vi "HOST.vi"() -> ()   [LabVIEW 2018]
uses:
  <instrlib>/niDMM/nidmm.llb/niDMM Function.ctl
  <instrlib>/niDMM/nidmm.llb/niDMM Resolution in Digits.ctl
  <instrlib>/niDMM/nidmm.llb/niDMM Configure Measurement Digits.vi
panel:
  in  "ЛОГИ":path=path "D:/NI LabVIEW/20.089_(KMKS_2)/LOGS"
  out "T(t)":dbl(graph)=398.0450506439805
  out "3ph P(t)":dbl(graph)
  out "3ph power, V":dbl=2.1649482628491312e-07 format="%#.5f"
  out "Temp, °C":dbl caption="Measurement" format="%.5f"
  out "Amps":dbl caption="Measurement" format="%.5f"
  out "Volts":dbl caption="Measurement" format="%.5f"
  out "Volts (Temp)":dbl caption="Measurement" format="%.5f"
  out "Power, V":dbl=7.216494209497104e-08 format="%#.5f"
  in  "Stop":bool
  in  "Temp Range\n(Volts)":dbl=2.0 format="%.2p"
  out "Out of Range (I)":bool caption="Signal Out of Range"
  in  "I":refnum<k15>="PXI1Slot5"
  in  "Range (Amps)":dbl=1.0 format="%.2p"
  out "Out of Range (V)":bool caption="Signal Out of Range"
  in  "U":refnum<k15>="PXI1Slot4"
  in  "Range (Volts)":dbl=2.0 format="%.2p"
  out "Out of Range (V, Temp)":bool caption="Signal Out of Range"
  in  "Temp":refnum<k15>="PXI1Slot3_4"
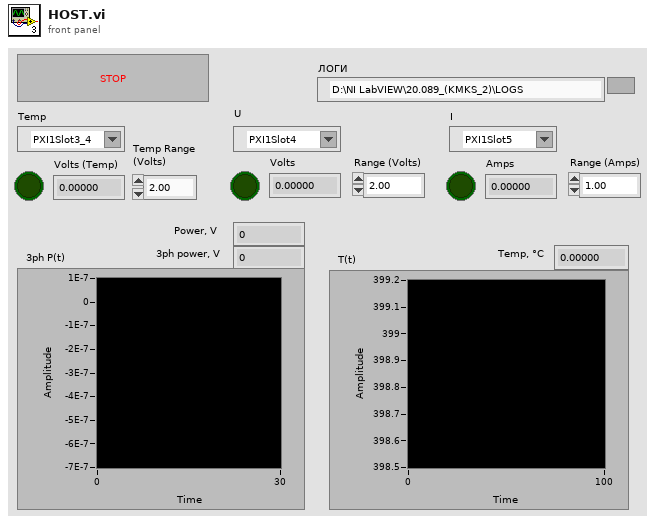
[diagram p1: front panel]
types:
  T1 = enum16{"open", "replace", "create", "open or create", "replace or create", "replace or create with confirmation"}
  T2 = typedef "niDMM Function.ctl" = enum16{"DC Volts", "AC Volts", "DC Current", "AC Current", "2-wire Resistance", "4-wire Resistance", "Diode", "Frequency", "Period", "AC Volts DC Coupled", "Capacitance", "Inductance", "Temperature"}
  T3 = typedef "niDMM Resolution in Digits.ctl" = dbl
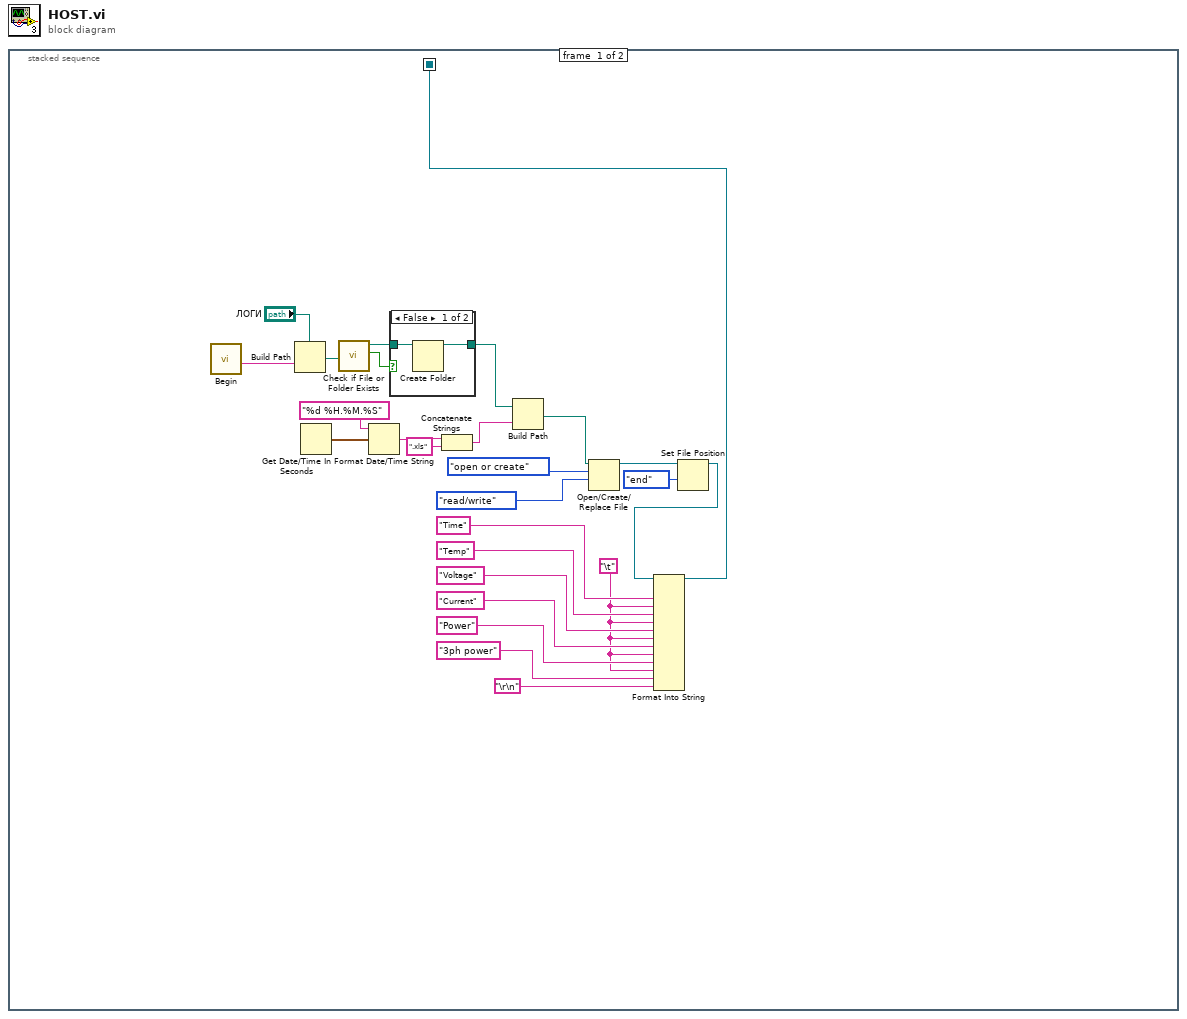
[diagram p0: block diagram]
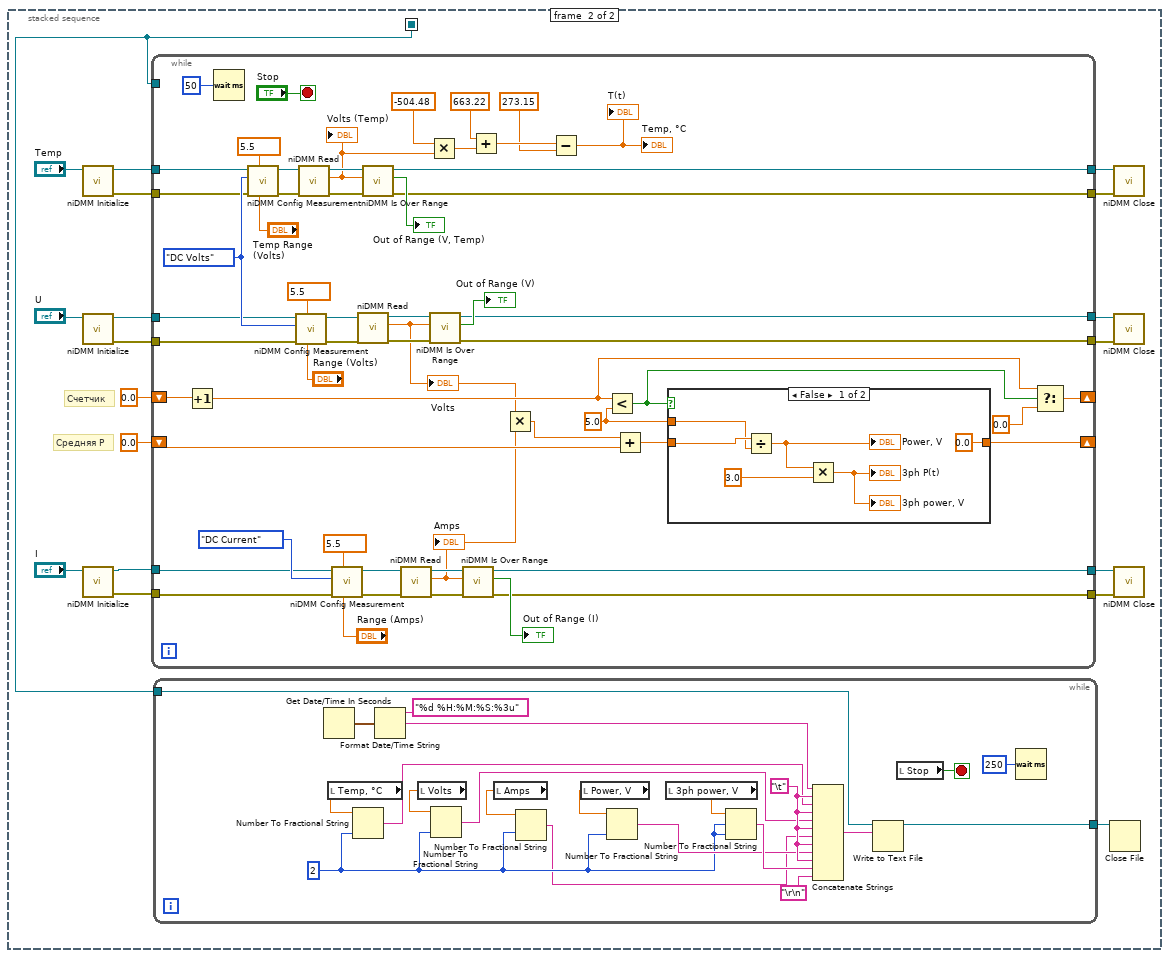
[diagram p3: hidden frame]
diagram:
  n1 = stacked-sequence {
    seq-local: [w3 _] -> [_ w31]
    frame #0 {
      w9 = "\t"
      n2 = call "Begin.vi"() -> ("Образец № 2"=w1:string)  [unwired: 8 in]
      n3 = Build Path(base path="ЛОГИ", name or relative path=w1) -> (appended path=w26:path)
      n4 = Get Date/Time In Seconds() -> (seconds since 1Jan1904=w22:timestamp)
      n5 = call <vilib>:"Check if File or Folder Exists.vi"("path"=w26) -> ("file or folder exists?"=w25:bool, "dup path"=w24:path)  [unwired: 8 in, 1 out]
      n6 = Format Date/Time String(time format string (%c)="%d %H.%M.%S", seconds (now)=w22) -> (date/time string=w21:string)  [unwired: 1 in]
      n7 = case shown="False" w25 {
        tunnel: w24 -> [w28 w29]
        tunnel: [w27 w29] -> w23
        frame False {
          n8 = Create Folder(path (use dialog)=w28) -> (created path=w27:path)  [unwired: 2 in, 2 out]
        }
        frame True {
        }
      }
      n9 = Concatenate Strings(w21, ".xls" ("string")) -> (w18:string)
      n10 = Build Path(base path=w23, name or relative path=w18) -> (appended path=w15:path)
      n11 = Open/Create/Replace File(file path (use dialog)=w15, operation (0:open)=T1."open or create", access (0:read/write)=enum16{"read/write", "read-only", "write-only"}."read/write") -> (refnum out=w6:refnum<file>)  [unwired: 3 in, 2 out]
      n12 = Set File Position(refnum=w6, from (0:start)=enum16{"start", "end", "current"}."end") -> (refnum out=w4:refnum<file>)  [unwired: 2 in, 1 out]
      n13 = Format Into String(initial string=w4, "Time" ("string"), w9, "Temp" ("string"), w9, "Voltage" ("string"), w9, "Current" ("string"), w9, "Power" ("string"), w9, "3ph power" ("string"), "\r\n") -> (resulting string=w3:refnum<file>)  [unwired: 2 in, 1 out]
    }
    frame #1 {
      # "Счетчик"
      # "Средняя P"
      n14 = call <instrlib>:"niDMM Initialize.vi"("Instrument Descriptor"="Temp") -> ("error out"=w38:errorcluster, "instrument handle out"=w39:refnum<k15>)  [unwired: 9 in]
      n15 = call <instrlib>:"niDMM Initialize.vi"("Instrument Descriptor"="U") -> ("error out"=w40:errorcluster, "instrument handle out"=w41:refnum<k15>)  [unwired: 9 in]
      n16 = call <instrlib>:"niDMM Initialize.vi"("Instrument Descriptor"="I") -> ("error out"=w34:errorcluster, "instrument handle out"=w35:refnum<k15>)  [unwired: 9 in]
      n17 = while {
        tunnel: [w103] -> w45
        tunnel: [w102] -> w44
        tunnel: [w101] -> w43
        tunnel: [w100] -> w42
        tunnel: w41 -> [w97]
        tunnel: w40 -> [w96]
        tunnel: w39 -> [w95]
        tunnel: w38 -> [w94]
        shift-right: [w83] -> _
        shift-left: 0.0 -> [w91]
        shift-right: [w84] -> _
        shift-left: 0.0 -> [w85]
        tunnel: w35 -> [w90]
        tunnel: w34 -> [w89]
        tunnel: [w88] -> w33
        tunnel: [w87] -> w32
        tunnel: w31 -> [_]
        stop <- "Stop" stop-if-true
        w70 = 5.0 ("y")
        w106 = T3 5.5 items=["3 1/2"=3.5, "4 1/2"=4.5, "5 1/2"=5.5, "6 1/2"=6.5, "7 1/2"=7.5] ("Resolution in Digits 3")
        w105 = T3 5.5 items=["3 1/2"=3.5, "4 1/2"=4.5, "5 1/2"=5.5, "6 1/2"=6.5, "7 1/2"=7.5] ("Resolution in Digits 2")
        w104 = T3 5.5 items=["3 1/2"=3.5, "4 1/2"=4.5, "5 1/2"=5.5, "6 1/2"=6.5, "7 1/2"=7.5] ("Resolution in Digits")
        w99 = niDMM_Function."DC Volts" ("Function")
        n18 = Increment(x=w91) -> (x+1=w79:dbl)
        n19 = Wait (ms)(milliseconds to wait=u32 50) -> ()  [unwired: 1 out]
        n20 = call-poly <instrlib>:"niDMM Config Measurement.vi"("Range"="Temp Range\n(Volts)", "Resolution in Digits"=w104, "error in (no error)"=w94, "Function"=w99, "instrument handle"=w95) -> ("error out"=w120:errorcluster, "instrument handle out"=w119:refnum<k15>)  [unwired: 5 in]
        n21 = call-poly <instrlib>:"niDMM Config Measurement.vi"("Range"="Range (Volts)", "Resolution in Digits"=w105, "error in (no error)"=w96, "Function"=w99, "instrument handle"=w97) -> ("error out"=w122:errorcluster, "instrument handle out"=w121:refnum<k15>)  [unwired: 5 in]
        n22 = call <instrlib>:"niDMM Read.vi"("error in (no error)"=w120, "instrument handle"=w119) -> ("error out"=w109:errorcluster, "Measurement"=w93:dbl, "instrument handle out"=w108:refnum<k15>)  [unwired: 7 in]
        "Volts (Temp)" <- w93
        n23 = call-poly <instrlib>:"niDMM Config Measurement.vi"("Range"="Range (Amps)", "Resolution in Digits"=w106, "error in (no error)"=w89, "Function"=niDMM_Function."DC Current", "instrument handle"=w90) -> ("error out"=w124:errorcluster, "instrument handle out"=w123:refnum<k15>)  [unwired: 5 in]
        n24 = call <instrlib>:"niDMM Read.vi"("error in (no error)"=w122, "instrument handle"=w121) -> ("error out"=w113:errorcluster, "Measurement"=w72:dbl, "instrument handle out"=w112:refnum<k15>)  [unwired: 7 in]
        "Volts" <- w72
        n25 = call <instrlib>:"niDMM Is Over Range.vi"("error in (no error)"=w109, "Measurement"=w93, "instrument handle"=w108) -> ("error out"=w102:errorcluster, "Over Range?"=→"Out of Range (V, Temp)":bool, "instrument handle out"=w103:refnum<k15>)  [unwired: 6 in]
        n26 = call <instrlib>:"niDMM Read.vi"("error in (no error)"=w124, "instrument handle"=w123) -> ("error out"=w117:errorcluster, "Measurement"=w71:dbl, "instrument handle out"=w116:refnum<k15>)  [unwired: 7 in]
        "Amps" <- w71
        n27 = Multiply(x=-504.48, y=w93) -> (x*y=w78:dbl)
        n28 = call <instrlib>:"niDMM Is Over Range.vi"("error in (no error)"=w113, "Measurement"=w72, "instrument handle"=w112) -> ("error out"=w100:errorcluster, "Over Range?"=→"Out of Range (V)":bool, "instrument handle out"=w101:refnum<k15>)  [unwired: 6 in]
        n29 = call <instrlib>:"niDMM Is Over Range.vi"("error in (no error)"=w117, "Measurement"=w71, "instrument handle"=w116) -> ("error out"=w87:errorcluster, "Over Range?"=→"Out of Range (I)":bool, "instrument handle out"=w88:refnum<k15>)  [unwired: 6 in]
        n30 = Add(x=663.22, y=w78) -> (x+y=w76:dbl)
        n31 = Multiply(x=w72, y=w71) -> (x*y=w81:dbl)
        n32 = Subtract(x=w76, y=273.15) -> (x-y=→"Temp, °C" →"T(t)":dbl)
        n33 = Less?(x=w79, y=w70) -> (x < y?=w80:bool)
        n34 = Add(x=w81, y=w85) -> (x+y=w86:dbl)
        n35 = case shown="False" w80 {
          tunnel: [0.0 w132] -> w84
          tunnel: w86 -> [w131 w132]
          tunnel: w70 -> [w127 _]
          frame False {
            n36 = Divide(x=w131, y=w127) -> (x/y=w128:dbl)
            "Power, V" <- w128
            n37 = Multiply(x=w128, y=3.0) -> (x*y=→"3ph P(t)" →"3ph power, V":dbl)
          }
          frame True {
          }
        }
        n38 = Select(t=w79, s=w80, f=0.0) -> (s? t:f=w83:dbl)
      }
      n39 = while {
        tunnel: w31 -> [w49]
        tunnel: [w67] -> w30
        stop <- w68 stop-if-true
        w65 = "\t"
        w59 = 2
        n40 = Get Date/Time In Seconds() -> (seconds since 1Jan1904=w52:timestamp)
        n41 = local read "Temp, °C"() -> (w53:dbl)
        n42 = Number To Fractional String(number=w53, precision (6)=w59) -> (F-format string=w60:string)  [unwired: 2 in]
        n43 = Format Date/Time String(time format string (%c)="%d %H:%M:%S:%3u", seconds (now)=w52) -> (date/time string=w50:string)  [unwired: 1 in]
        n44 = local read "Volts"() -> (w56:dbl)
        n45 = Number To Fractional String(number=w56, precision (6)=w59) -> (F-format string=w61:string)  [unwired: 2 in]
        n46 = local read "Amps"() -> (w58:dbl)
        n47 = Number To Fractional String(number=w58, precision (6)=w59) -> (F-format string=w57:string)  [unwired: 2 in]
        n48 = local read "Power, V"() -> (w55:dbl)
        n49 = Number To Fractional String(number=w55, precision (6)=w59) -> (F-format string=w62:string)  [unwired: 2 in]
        n50 = local read "3ph power, V"() -> (w54:dbl)
        n51 = Number To Fractional String(number=w54, width (-)=w59, precision (6)=w59) -> (F-format string=w63:string)  [unwired: 1 in]
        n52 = Concatenate Strings(w50, w65, w60, w65, w61, w65, w57, w65, w62, w65, w63, "\r\n") -> (w66:string)
        n53 = Write to Text File(file (use dialog)=w49, text=w66) -> (refnum out=w67:refnum<file>)  [unwired: 2 in, 2 out]
        n54 = local read "Stop"() -> (w68:bool)
        n55 = Wait (ms)(milliseconds to wait=u32 250) -> ()  [unwired: 1 out]
      }
      n56 = Close File(refnum=w30) -> ()  [unwired: 1 in, 2 out]
      n57 = call <instrlib>:"niDMM Close.vi"("error in (no error)"=w44, "instrument handle"=w45) -> ()  [unwired: 9 in, 1 out]
      n58 = call <instrlib>:"niDMM Close.vi"("error in (no error)"=w42, "instrument handle"=w43) -> ()  [unwired: 9 in, 1 out]
      n59 = call <instrlib>:"niDMM Close.vi"("error in (no error)"=w32, "instrument handle"=w33) -> ()  [unwired: 9 in, 1 out]
    }
  }
